vi "GenerateCode.vi"(1 "Terms":T1[](array[typedef]), 3 "Diagram":refnum<vi>, 5 "XRef":refnum<vi>, 6 "State In":T4={"Input Type"=variant(dbl 0.0), "Error"={"status"=FALSE, "code"=0, "source"=""}}) -> (0 "Generated Code?":bool, 2 "State Out":T4={"Input Type"=variant(dbl 0.0), "Error"={"status"=FALSE, "code"=0, "source"=""}}, 4 "Reply":string[](array[string]))   [LabVIEW 2015, in "Destroy-Signals.xnode"]
doc: "This ability VI is called when it is time to define the execution behavior of your XNode via LabVIEW's scripting API. This VI is only called when you have previously informed LabVIEW that you need to script through a GenerateCode reply. Diagram is a reference to a diagram of a temporary VI. This diagram contains exactly one front panel terminal for each terminal of your XNode. Terms is an array of pairs of Term IDs and terminal references. LabVIEW will copy code scripted into this diagram into your XNode and connect everything to the correct terminals. The front panel terminals that are on this diagram are special in that they can only be on the top level diagram.\n \n Generate Code? is used to tell LabVIEW whether or not you want to copy the scripted diagram over. If there is an error and you wish not to commit the changes, then the old XNode behavior will be left unchanged. If you set Generate Code? to false, then this VI will be called again next time type propagation is run. Otherwise, it will not be called until you indicate that it should be through the reply on another ability VI.\n \n Because the diagram you are scripting into is separate from the VI containing the XNode instance, type propagation and the data manager will run on the temporary VI after each scripting call.\n \n You should not use the Copy scripting method to move code into the temporary VI. This will adversely affect the user's clipboard. You should use the Move scripting method instead.\n\nDefault behavior: None.\n\nThis ability does not provide UI and OS messages are not handled.\n\nSee also: ModifyCode"
uses:
  Destroy-Signals.xnode
  State.ctl
  <vilib>/XNodeSupport/XNodeTermIDPair.ctl
  <vilib>/XNodeSupport/XNodeTermRef.ctl
  <vilib>/XNodeSupport/XNodeString.ctl
  <vilib>/LV-Scripting/LV-Scripting.lvlib
  <vilib>/XNodeSupport/NI_XNodeSupport.lvlib
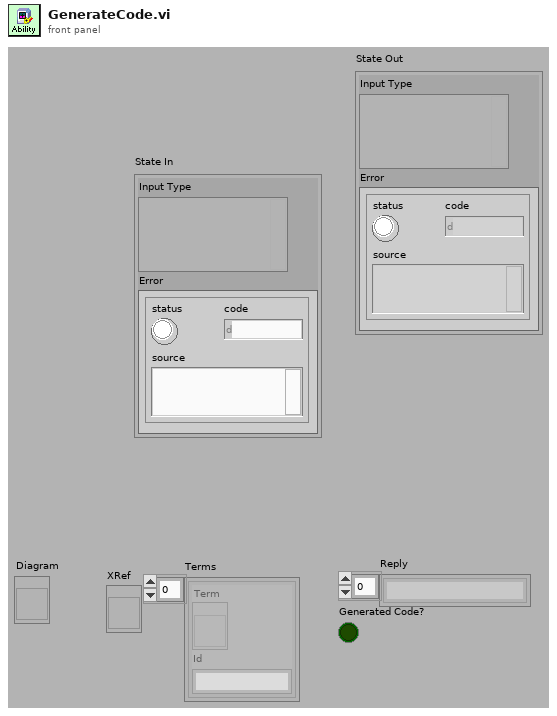
[diagram p1: front panel]
types:
  T1 = typedef "NI_XNodeSupport.lvlib/XNodeTermIDPair.ctl" = cluster{"Term":T2, "Id":T3}
  T2 = typedef "NI_XNodeSupport.lvlib/XNodeTermRef.ctl" = refnum<vi>
  T3 = typedef "NI_XNodeSupport.lvlib/XNodeString.ctl" = string
  T4 = typedef "Destroy-Signals.xnode/State.ctl" = cluster{"Input Type":variant, "Error":errorcluster}
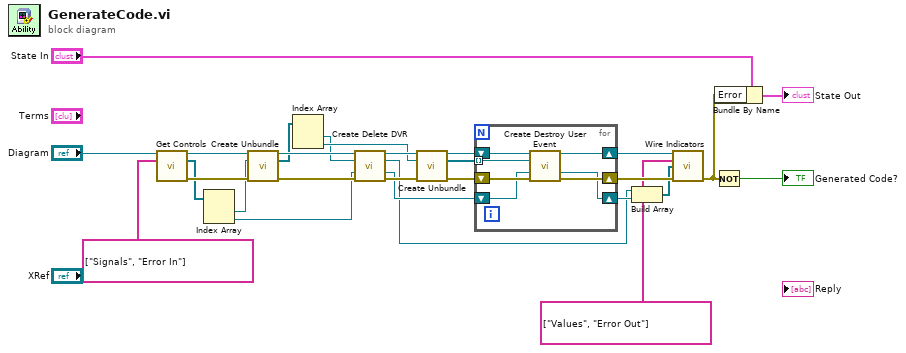
[diagram p0: block diagram]
diagram:
  n1 = call <vilib>:"Get Controls.vi"("Diagram in"="Diagram", "Control Names"=string[] ["Signals", "Error In"]) -> ("Diagram out"=w26:refnum<vi>, "Control Terminals"=w16:refnum<vi>[], "error out"=w25:errorcluster)  [unwired: 11 in]
  n2 = Index Array(array=w16) -> (element #1=w15:refnum<vi>, element #2=w14:refnum<vi>)  [unwired: 2 in]
  n3 = call <vilib>:"Create Unbundle.vi"("Diagram in"=w26, "input cluster"=w15, "error in (no error)"=w25) -> ("Diagram out"=w24:refnum<vi>, "Outputs"=w13:refnum<vi>[], "error out"=w23:errorcluster)  [unwired: 10 in]
  n4 = Index Array(array=w13) -> (element #1=w3:refnum<vi>, element #2=w4:refnum<vi>)  [unwired: 2 in]
  n5 = call <vilib>:"Create Delete DVR.vi"("Diagram in"=w24, "data value reference"=w3, 9:"error in (no error)"=w14, 11:"error in (no error)"=w23) -> ("Diagram out"=w22:refnum<vi>, "data value"=w1:refnum<vi>, 10:"error out"=w2:refnum<vi>, 15:"error out"=w21:errorcluster)  [unwired: 8 in]
  n6 = call <vilib>:"Create Unbundle.vi"("Diagram in"=w22, "input cluster"=w4, "error in (no error)"=w21) -> ("Diagram out"=w20:refnum<vi>, "Outputs"=w12:refnum<vi>[], "error out"=w19:errorcluster)  [unwired: 10 in]
  n7 = for {
    shift-right: [w33] -> w17
    shift-left: w19 -> [w34]
    shift-right: [w32] -> w18
    shift-left: w20 -> [w35]
    shift-right: [w29] -> w10
    shift-left: w2 -> [w31]
    tunnel: w12 -> [w30] mode=indexing
    n8 = call <vilib>:"Create Destroy User Event.vi"("Diagram in"=w35, "user event"=w30, "error in"=w31, "error in (no error)"=w34) -> ("Diagram out"=w32:refnum<vi>, 10:"error out"=w29:refnum<vi>, 15:"error out"=w33:errorcluster)  [unwired: 9 in]
  }
  n9 = Build Array(w1, w10) -> (w9:refnum<vi>[])
  n10 = call <vilib>:"Wire Indicators.vi"("Diagram in"=w18, "Indicator Names"=string[] ["Values", "Error Out"], "Outputs"=w9, "error in (no error)"=w17) -> ("error out"=w6:errorcluster)  [unwired: 10 in, 1 out]
  n11 = Not(x=w6) -> (.not. x?=→"Generated Code?":bool)
  n12 = Bundle By Name(cluster="State In", "Error"=w6) -> (→"State Out":T4)
